vi "Report build (SubVI).vi"(0 "Full/Fails":string(combo)="Full", 1 "Operator":string, 2 "Original ATR Ref":refnum<vi>, 3 "GeneralResult-Pass(T)Fail(F)":bool, 4 "Header Array":string[][](array[string]), 5 "error in (no error)":errorcluster, 6 "report file path":path) -> (19 "error out":errorcluster)   [LabVIEW 2017]
uses:
  <vilib>/Utility/miscctls.llb/LVRowAndColumnUnsignedTypeDef.ctl
  <vilib>/Utility/NIReport.llb/Append Image to Report (path wrap).vi
  <vilib>/Utility/NIReport.llb/Append Text Table to Report (wrap).vi
  <vilib>/Utility/NIReport.llb/Append Report Text (str wrap).vi
  <vilib>/Utility/NIReport.llb/NI_report.lvclass
  <vilib>/Utility/NIReport.llb/Word/NI_Word.lvclass
  <vilib>/addons/_office/NI_ReportGenerationToolkit.lvlib
panel:
  in  "ATR":string[][](table)=[["Test Communication", "-", "-", "-", "-", ""], ["Set S/N", "-", "-", "-", "-", ""], ["Set Board Number", "-", "-", "-", "-", ""], [" ", "", "", "", "", ""], ["Test Communication", "-", "-", "-", "-", ""], ["Get S/N", "-", "-", "-", "", ""], ["Get Board Number", "-", "-", "-", "", ""], ["Get FW", "-", "-", "-", "", ""], ["Enable Motor", "", "", "", "", ""], ["Small position command", "", "", "", "", ""], ["Measure delta", "", "", "", "", ""], ["Velocity command", "", "", "", "", ""]]
  in  "Pass  Button":bool
  in  "Fail  Button":bool
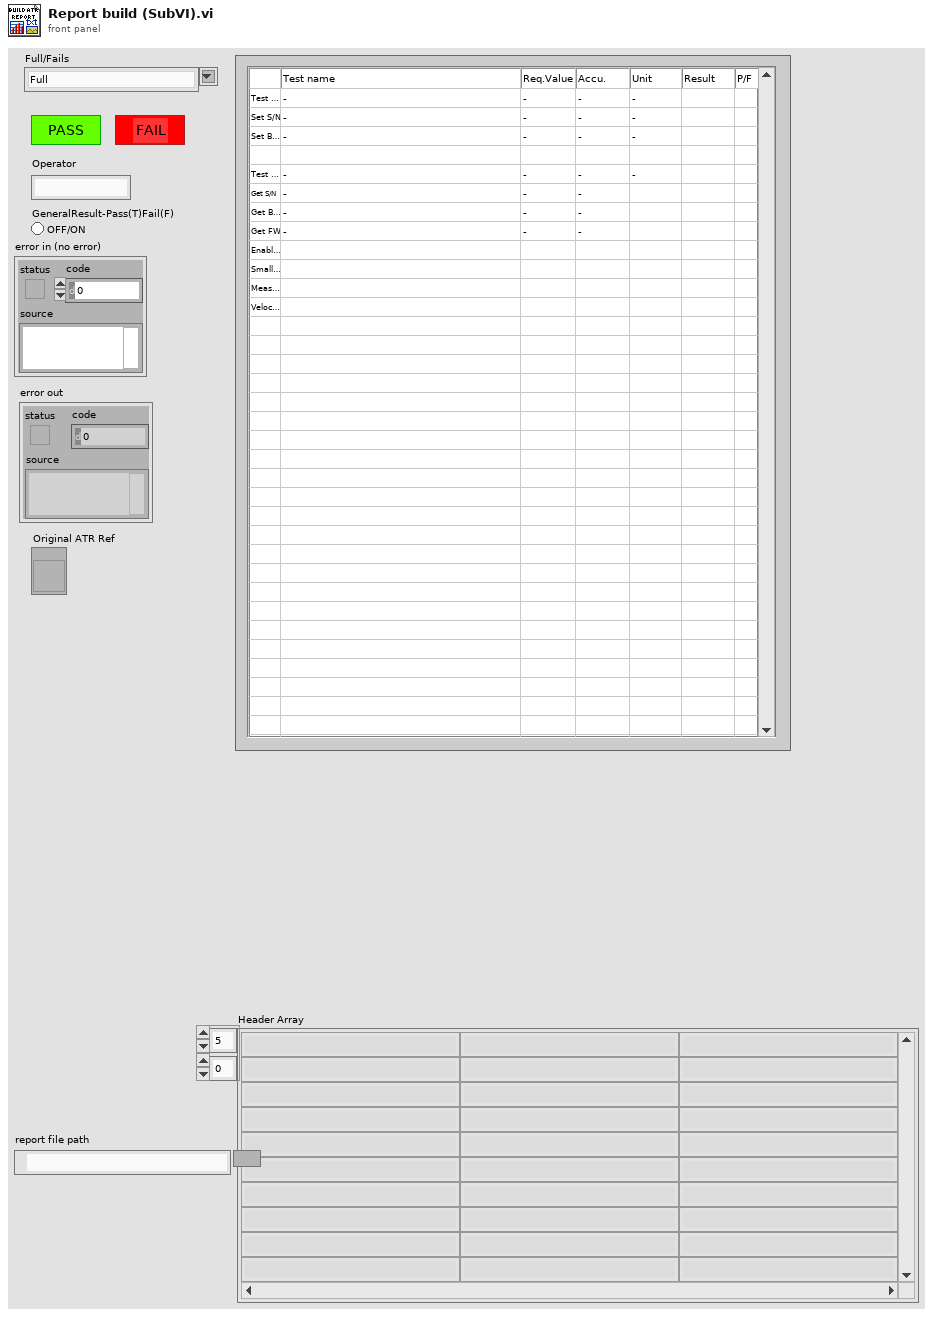
[diagram p1: front panel]
types:
  T1 = cluster{"top":dbl, "left":dbl, "right":dbl, "bottom":dbl}
  T2 = cluster{"alignment":enum16{"Left", "Centered", "Right", "Justify"}, "left":dbl, "right":dbl, "special":enum16{"(none)", "First line", "Hanging"}, "by":dbl, "before":dbl, "after":dbl, "line spacing":enum16{"Single", "1,5 lines", "Double", "At least", "Exactly", "Multiple"}, "at":dbl}
  T3 = enum16{"maximized", "minimized", "normal", "no change"}
  T4 = enum16{"Standard Report", "HTML", "Word", "Excel"}
  T5 = typedef "LVRowAndColumnUnsignedTypeDef.ctl" = cluster{"Row":u32, "Column":u32}
  T6 = typedef "LVFontTypeDef.ctl" = cluster{"Font Name":string, "Size":u16, "Bold":bool, "Italic":bool, "Underline":bool, "Strikeout":bool, "Color":u32}
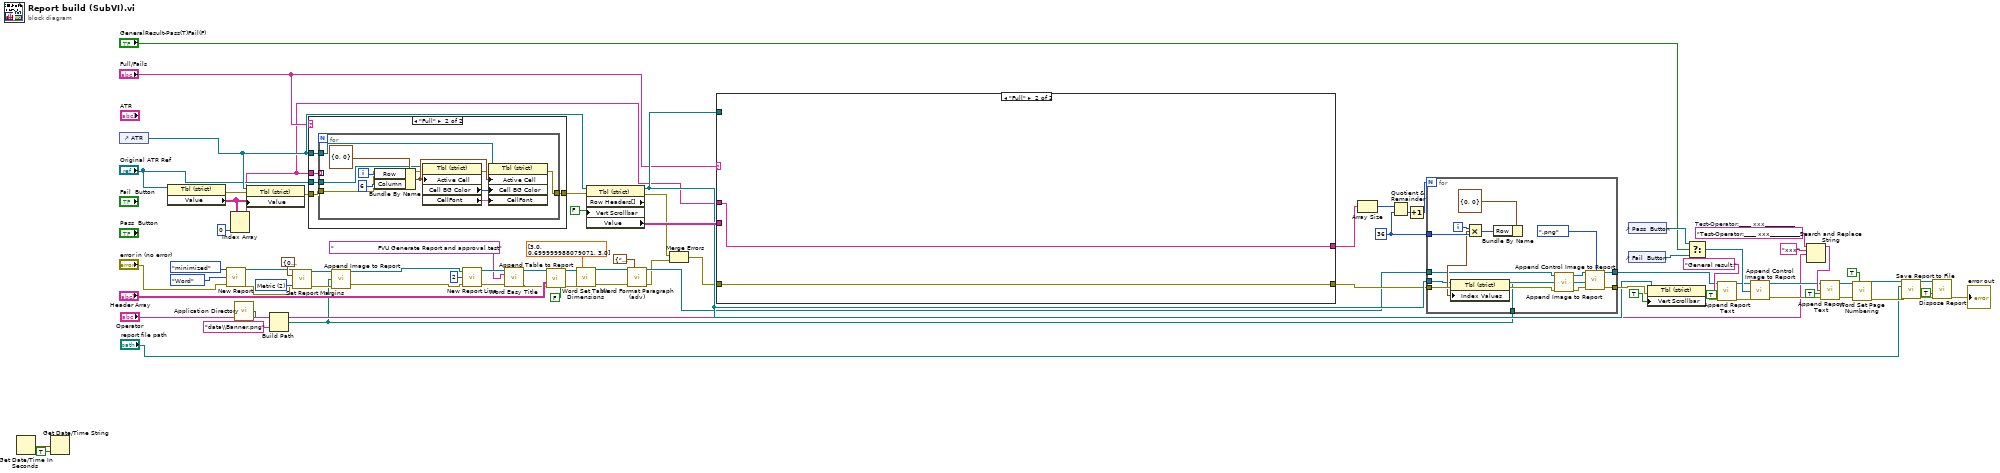
[diagram p0: block diagram]
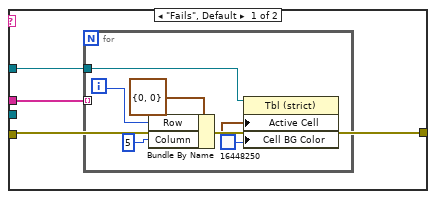
[diagram p2: hidden frame]
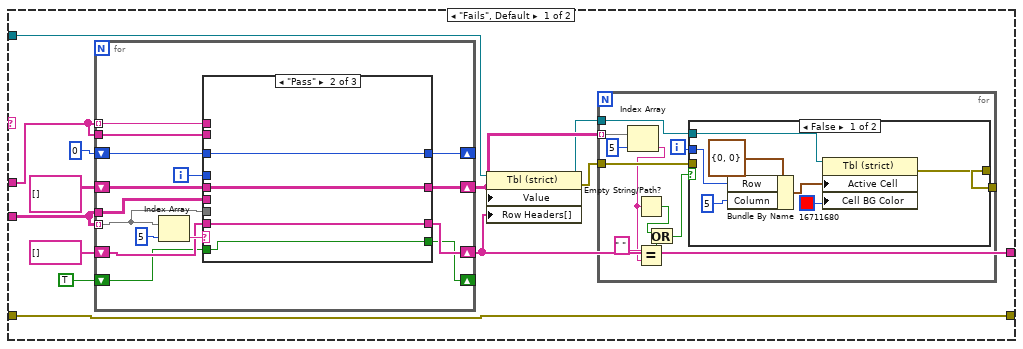
[diagram p3: hidden frame]
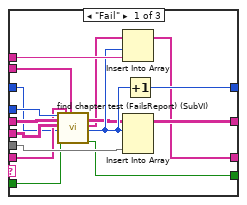
[diagram p5: hidden frame]
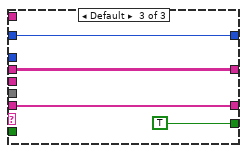
[diagram p6: hidden frame]
diagram:
  w10 = u16 2 items=["Default", "US", "Metric"] ("measurement system (default)")
  w64 = "Test-Operator:____ xxx__________"  # Test-Operator:____ xxx__________
  w77 = 36 ("y")
  n1 = Get Date/Time In Seconds() -> (seconds since 1Jan1904=w23:timestamp)
  n2 = Get Date/Time String(seconds (now)=w23, want seconds? (F)=TRUE) -> ()  [unwired: 1 in, 2 out]
  n3 = control-ref of="ATR"() -> (w69:refnum<vi>)
  n4 = property class="Tbl (strict)"(reference="Original ATR Ref") -> (error out=w34:errorcluster, "Value"=w14:string[][])  [unwired: 1 in, 1 out]
  n5 = call <vilib>:"New Report.vi"("window state (normal)"=T3."minimized", "report type"=T4."Word", "error in (no error)"="error in (no error)") -> ("report out"=w5:refnum<class "NI_report.lvclass">, "error out"=w4:errorcluster)  [unwired: 11 in]
  n6 = Index Array(array=w14, index (col)=0 ("disabled index (col)")) -> (element=w12:string[])  [unwired: 1 in]
  n7 = call <vilib>:"Application Directory.vi"() -> ("Application Directory"=w9:path)
  n8 = property class="Tbl (strict)"(reference=w69, error in=w34, "Value"=w14) -> (error out=w67:errorcluster)  [unwired: 1 out]
  n9 = Build Path(base path=w9, name or relative path="data\\Banner.png") -> (appended path=w1:path)
  n10 = call-dynamic "Set Report Margins.vi"("report in"=w5, "margins (1.00)"=T1 {"top"=0.1, "left"=2.5, "right"=1.0, "bottom"=0.75}, "measurement system (default)"=w10, "error in (no error)"=w4) -> ("report out"=w7:refnum<class "NI_report.lvclass">, "error out"=w6:errorcluster)  [unwired: 9 in, 1 out]
  n11 = case shown="\"Full\"" "Full/Fails" {
    tunnel: w69 -> [w82 w95]
    tunnel: "Original ATR Ref" -> [_ w94]
    tunnel: [w84 w93] -> w68
    tunnel: w67 -> [w84 w92]
    tunnel: w12 -> [w83 w91]
    frame "Fails", Default {
      n12 = for {
        tunnel: w83 -> [_] mode=indexing
        tunnel: w82 -> [w85]
        i -> [w90]
        n13 = Bundle By Name(cluster=T5 {"Row"=0, "Column"=0} ("Index Values"), "Row"=w90, "Column"=u32 5) -> (w88:T5)
        n14 = property class="Tbl (strict)"(reference=w85, "Active Cell"=w88, "Cell BG Color"=u32 16448250) -> ()  [unwired: 1 in, 2 out]
      }
    }
    frame "Full" {
      n15 = for {
        tunnel: w95 -> [w100]
        tunnel: w94 -> [w99]
        tunnel: [w98] -> w93
        tunnel: w92 -> [w96]
        tunnel: w91 -> [_] mode=indexing
        i -> [w101]
        n16 = Bundle By Name(cluster=T5 {"Row"=0, "Column"=0} ("Index Values"), "Row"=w101, "Column"=u32 6) -> (w103:T5)
        n17 = property class="Tbl (strict)"(reference=w99, error in=w96, "Active Cell"=w103) -> (error out=w97:errorcluster, "Cell BG Color"=w106:u32, "CellFont"=w105:T6)  [unwired: 1 out]
        n18 = property class="Tbl (strict)"(reference=w100, error in=w97, "Active Cell"=w103, "Cell BG Color"=w106, "CellFont"=w105) -> (error out=w98:errorcluster)  [unwired: 1 out]
      }
    }
  }
  n19 = call-poly <vilib>:"Append Image to Report.vi"("report in"=w7, "path or URL of image"=w1, "error in (no error)"=w6) -> ("report out"=w3:refnum<class "NI_report.lvclass">, "error out"=w2:errorcluster)  [unwired: 9 in, 2 out]
  n20 = call-dynamic "New Report Line.vi"("report in"=w3, "number of lines (1)"=2, "error in (no error)"=w2) -> ("report out"=w20:refnum<class "NI_report.lvclass">, "error out"=w19:errorcluster)  [unwired: 11 in]
  n21 = call <vilib>:"Word Easy Title.vi"("report in"=w20, "title"="                      FVU Generate Report and approval test" ("text"), "error in (no error)"=w19) -> ("report out"=w17:refnum<class "NI_report.lvclass">, "error out"=w18:errorcluster)  [unwired: 10 in, 1 out]
  n22 = call-poly <vilib>:"Append Table to Report.vi"("report in"=w17, "text data"="Header Array", "error in (no error)"=w18, "show grid lines (YES)"=FALSE) -> ("report out"=w47:refnum<class "NI_report.lvclass">, "error out"=w46:errorcluster)  [unwired: 8 in, 2 out]
  n23 = call <vilib>:"Word Set Table Dimensions.vi"("report in"=w47, "table column widths"=sgl[] [3.0, 0.7, 3.0], "error in (no error)"=w46) -> ("report out"=w41:refnum<class "NI_report.lvclass">, "error out"=w40:errorcluster)  [unwired: 11 in]
  n24 = property class="Tbl (strict)" props=["Row Headers[]", "Vert Scrollbar", "Value"](reference=w69, error in=w68, "Vert Scrollbar"=FALSE ("Visible Items:Vertical Scrollbar Visible")) -> (reference out=w71:refnum<vi>, error out=w37:errorcluster, "Value"=w75:string[][])  [unwired: 1 out]
  n25 = call <vilib>:"Word Format Paragraph (adv).vi"("report in"=w41, "indent and spacing"=T2 {"alignment"=enum."Left", "left"=0.0, "right"=0.0, "special"=enum."(none)", "by"=0.0, "before"=0.0, "after"=0.0, "line spacing"=enum."Single", "at"=0.0}, "error in (no error)"=w40) -> ("report out"=w39:refnum<class "NI_report.lvclass">, "error out"=w36:errorcluster)  [unwired: 11 in]
  n26 = Merge Errors(w37, w36) -> (w35:errorcluster)
  n27 = case shown="\"Full\"" "Full/Fails" {
    tunnel: w35 -> [w118 w177]
    tunnel: w12 -> [w113 w178]
    tunnel: [w118 w177] -> w70
    tunnel: w75 -> [w114 _]
    tunnel: [w110 w178] -> w74
    tunnel: w71 -> [w111 _]
    frame "Fails", Default {
      n28 = for {
        tunnel: w114 -> [w146] mode=indexing
        shift-right: [w148] -> w109
        shift-left: string[][] [] -> [w150]
        shift-right: [w147] -> _
        shift-left: 0 -> [w149]
        tunnel: w113 -> [w144] mode=indexing
        shift-right: [w143] -> w110
        shift-left: string[] [] -> [w145]
        tunnel: w114 -> [w141]
        tunnel: w113 -> [w140]
        shift-right: [w138] -> _
        shift-left: TRUE -> [w139]
        i -> [w142]
        n29 = Index Array(array=w146, index=5) -> (element=w151:string)
        n30 = case shown="\"Pass\"" w151 {
          tunnel: w150 -> [w162 w171 w175]
          tunnel: w149 -> [w159 w172 w176]
          tunnel: [w168 w171 w175] -> w148
          tunnel: [w167 w172 w176] -> w147
          tunnel: w146 -> [w166 _ _]
          tunnel: w145 -> [w161 w170 w174]
          tunnel: w144 -> [w160 _ _]
          tunnel: [w165 w170 w174] -> w143
          tunnel: w142 -> [w163 _ _]
          tunnel: w141 -> [w164 _ _]
          tunnel: w140 -> [w155 _ _]
          tunnel: w139 -> [w154 w169 _]
          tunnel: [w153 w169 TRUE ("ToExecute? Out")] -> w138
          frame "Fail" {
            n31 = call "find chapter test (FailsReport) (SubVI).vi"("ForLoopIndex"=w163, "Fails ATR IN"=w162, "Full ATR"=w164, "FailsATR Index IN"=w159, "ToExecute?"=w154, "Fails ATR RowHeader IN"=w161, "Full ATR RowHeader"=w155) -> ("Fails ATR OUT"=w157:string[][], "Fails ATR RowHeader OUT"=w156:string[], "FailsATR Index OUT"=w158:i32, "ToExecute? Out"=w153:bool)  [unwired: 9 in]
            n32 = Insert Into Array(array=w156, index=w158, new element=w160) -> (w165:string[])
            n33 = Insert Into Array(array=w157, index (row)=w158, new element=w166) -> (w168:string[][])  [unwired: 1 in]
            n34 = Increment(x=w158) -> (x+1=w167:i32)
          }
          frame "Pass" {
          }
          frame Default {
          }
        }
      }
      n35 = property class="Tbl (strict)"(reference=w111, "Value"=w109, "Row Headers[]"=w110) -> (reference out=w107:refnum<vi>, error out=w108:errorcluster)  [unwired: 1 in]
      n36 = for {
        tunnel: [w128] -> _
        tunnel: w109 -> [w127] mode=indexing
        tunnel: w108 -> [w125]
        tunnel: w107 -> [w124]
        i -> [w129]
        n37 = Index Array(array=w127, index=5) -> (element=w121:string)
        n38 = Empty String/Path?(string/path=w121) -> (empty?=w123:bool)
        n39 = Equal?(x=" ", y=w121) -> (x = y?=w120:bool)
        n40 = Or(x=w123, y=w120) -> (x .or. y?=w119:bool)
        n41 = case shown="False" w119 {
          tunnel: w129 -> [w133 _]
          tunnel: [w132 w137] -> w128
          tunnel: w125 -> [_ w137]
          tunnel: w124 -> [w130 _]
          frame False {
            n42 = Bundle By Name(cluster=T5 {"Row"=0, "Column"=0} ("Index Values"), "Row"=w133, "Column"=u32 5) -> (w135:T5)
            n43 = property class="Tbl (strict)"(reference=w130, "Active Cell"=w135, "Cell BG Color"=u32 16711680) -> (error out=w132:errorcluster)  [unwired: 1 in, 1 out]
          }
          frame True {
          }
        }
      }
    }
    frame "Full" {
    }
  }
  n44 = Array Size(array=w74) -> (size(s)=w78:i32)
  n45 = Quotient & Remainder(x=w78, y=w77) -> (floor(x/y)=w79:i32)  [unwired: 1 out]
  n46 = Increment(x=w79) -> (x+1=w80:i32)
  n47 = for {
    N: w80 -> [_]
    tunnel: w77 -> [w191]
    tunnel: w39 -> [w181]
    tunnel: w70 -> [w188]
    tunnel: [w189] -> w72
    tunnel: w71 -> [w185]
    tunnel: [w184] -> w58
    tunnel: w1 -> [w179]
    i -> [w192]
    n48 = Multiply(x=w192, y=w191) -> (x*y=w193:i32)
    n49 = Bundle By Name(cluster=T5 {"Row"=0, "Column"=0} ("Index Values"), "Row"=w193) -> (w187:T5)
    n50 = property class="Tbl (strict)"(reference=w185, error in=w188, "Index Values"=w187) -> (reference out=w186:refnum<vi>, error out=w180:errorcluster)
    n51 = call-poly <vilib>:"Append Image to Report.vi"("report in"=w181, "path or URL of image"=w179, "error in (no error)"=w180) -> ("report out"=w182:refnum<class "NI_report.lvclass">, "error out"=w183:errorcluster)  [unwired: 9 in, 2 out]
    n52 = call-dynamic "Append Control Image to Report.vi"("report in"=w182, "image file type (.jpg)"=enum16{".jpg", ".png"}.".png" ("image file type(.jpg)"), "ctrl reference"=w186, "error in (no error)"=w183) -> ("report out"=w184:refnum<class "NI_report.lvclass">, "error out"=w189:errorcluster)  [unwired: 8 in, 2 out]
  }
  n53 = control-ref of="Fail  Button"() -> (w60:refnum<vi>)
  n54 = control-ref of="Pass  Button"() -> (w61:refnum<vi>)
  n55 = property class="Tbl (strict)"(reference=w71, error in=w72, "Vert Scrollbar"=TRUE ("Visible Items:Vertical Scrollbar Visible")) -> (error out=w56:errorcluster)  [unwired: 1 out]
  n56 = Select(t=w61, s="GeneralResult-Pass(T)Fail(F)", f=w60) -> (s? t:f=w62:refnum<vi>)
  n57 = call-poly <vilib>:"Append Report Text.vi"("report in"=w58, "text"="General result:", "append on new line? (F)"=TRUE, "error in (no error)"=w56) -> ("report out"=w54:refnum<class "NI_report.lvclass">, "error out"=w55:errorcluster)  [unwired: 8 in, 2 out]
  n58 = call-dynamic "Append Control Image to Report.vi"("report in"=w54, "ctrl reference"=w62, "error in (no error)"=w55) -> ("report out"=w53:refnum<class "NI_report.lvclass">, "error out"=w52:errorcluster)  [unwired: 9 in, 2 out]
  n59 = Search and Replace String(input string=w64, search string="xxx", replace string="Operator") -> (result string=w63:string)  [unwired: 5 in, 3 out]
  n60 = call-poly <vilib>:"Append Report Text.vi"("report in"=w53, "text"=w63, "append on new line? (F)"=TRUE, "error in (no error)"=w52) -> ("report out"=w31:refnum<class "NI_report.lvclass">, "error out"=w30:errorcluster)  [unwired: 8 in, 2 out]
  n61 = call <vilib>:"Word Set Page Numbering.vi"("report in"=w31, "include page x of n"=TRUE, "error in (no error)"=w30) -> ("report out"=w28:refnum<class "NI_report.lvclass">, "error out"=w29:errorcluster)  [unwired: 11 in]
  n62 = call-dynamic "Save Report to File.vi"("report in"=w28, "report file path"="report file path", "error in (no error)"=w29) -> ("report out"=w26:refnum<class "NI_report.lvclass">, "error out"=w27:errorcluster)  [unwired: 11 in]
  n63 = call-dynamic "Dispose Report.vi"("report in"=w26, "save changes? (F)"=TRUE, "error in (no error)"=w27) -> ("error out"=→"error out":errorcluster)  [unwired: 12 in]
